vi "Lifting Position Calculations.vi"(0 "Limit switch 4":bool, 1 "position":enum16{"0", "1", "2", "3", "4"}(ring), 5 "Limit switch 3":bool, 7 "Limit switch 2":bool, 9 "Limit switch 1":bool, 11 "Bottom Limit switch":bool) -> (6 "Direction":enum16{"stop", "up", "down"}(ring), 10 "current position":dbl)   [LabVIEW 2014]
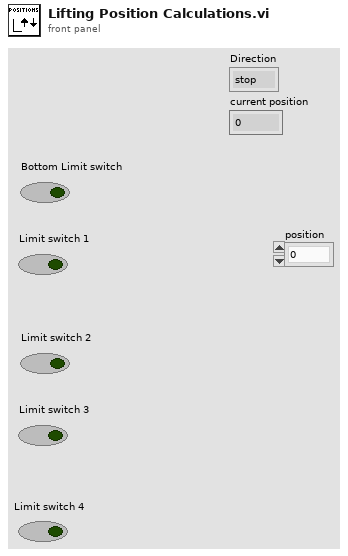
[diagram p1: front panel]
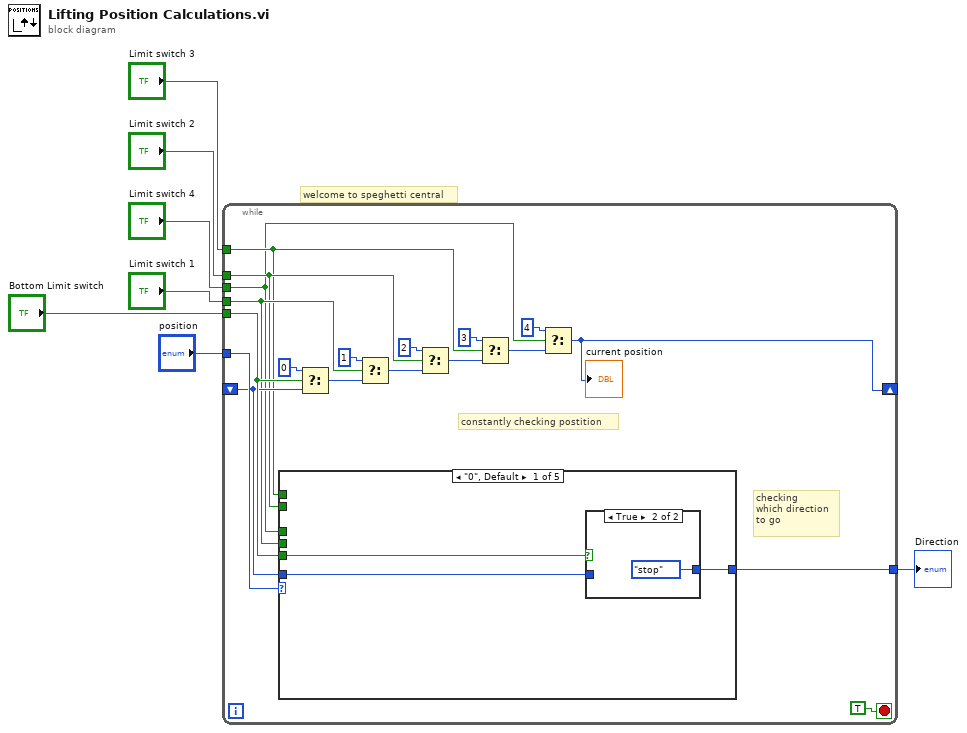
[diagram p0: block diagram]
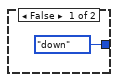
[diagram p2: hidden frame]
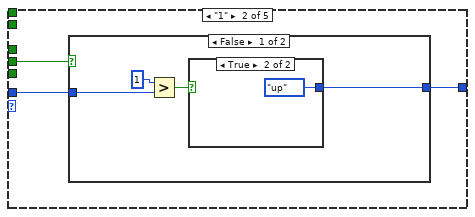
[diagram p3: hidden frame]
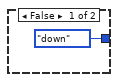
[diagram p4: hidden frame]
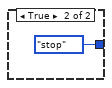
[diagram p5: hidden frame]
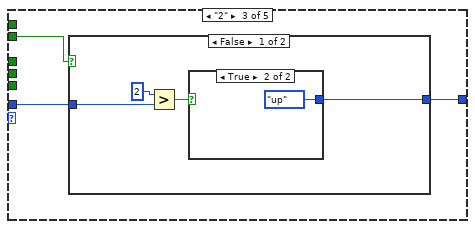
[diagram p6: hidden frame]
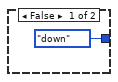
[diagram p7: hidden frame]
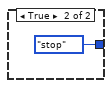
[diagram p8: hidden frame]
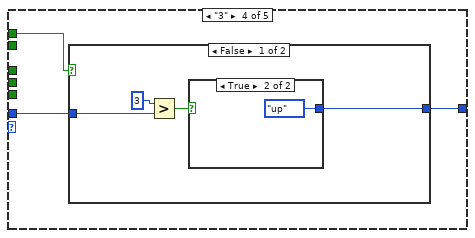
[diagram p9: hidden frame]
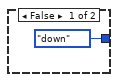
[diagram p10: hidden frame]
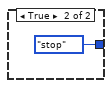
[diagram p11: hidden frame]
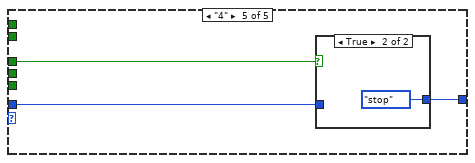
[diagram p12: hidden frame]
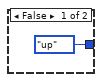
[diagram p13: hidden frame]
diagram:
  # "welcome to speghetti central"
  n1 = while {
    tunnel: "position" -> [w26]
    tunnel: [w25] -> w6
    tunnel: "Bottom Limit switch" -> [w13]
    tunnel: "Limit switch 1" -> [w11]
    tunnel: "Limit switch 2" -> [w10]
    tunnel: "Limit switch 3" -> [w9]
    tunnel: "Limit switch 4" -> [w8]
    shift-right: [w14] -> _
    shift-left: _ -> [w12]
    stop <- TRUE stop-if-true
    # "checking\nwhich direction\nto go"
    # "constantly checking postition"
    n2 = case shown="\"0\", Default" w26 {
      tunnel: [w29 w34 w44 w54 w64] -> w25
      tunnel: w13 -> [w28 _ _ _ _]
      tunnel: w11 -> [_ w33 _ _ _]
      tunnel: w10 -> [_ _ w43 _ _]
      tunnel: w9 -> [_ _ _ w53 _]
      tunnel: w8 -> [_ _ _ _ w63]
      tunnel: w12 -> [w27 w32 w42 w52 w62]
      frame "0", Default {
        n3 = case shown="True" w28 {
          tunnel: [enum16{"stop", "up", "down"}."down" ("Direction") enum16{"stop", "up", "down"}."stop" ("Direction")] -> w29
          tunnel: w27 -> [_ _]
          frame False {
          }
          frame True {
          }
        }
      }
      frame "1" {
        n4 = case shown="False" w33 {
          tunnel: [w38 enum16{"stop", "up", "down"}."stop" ("Direction")] -> w34
          tunnel: w32 -> [w35 _]
          frame False {
            n5 = Greater?(x=1, y=w35) -> (0:w36:bool)
            n6 = case shown="True" w36 {
              tunnel: [enum16{"stop", "up", "down"}."down" ("Direction") enum16{"stop", "up", "down"}."up" ("Direction")] -> w38
              frame False {
              }
              frame True {
              }
            }
          }
          frame True {
          }
        }
      }
      frame "2" {
        n7 = case shown="False" w43 {
          tunnel: [w48 enum16{"stop", "up", "down"}."stop" ("Direction")] -> w44
          tunnel: w42 -> [w45 _]
          frame False {
            n8 = Greater?(x=2, y=w45) -> (0:w47:bool)
            n9 = case shown="True" w47 {
              tunnel: [enum16{"stop", "up", "down"}."down" ("Direction") enum16{"stop", "up", "down"}."up" ("Direction")] -> w48
              frame False {
              }
              frame True {
              }
            }
          }
          frame True {
          }
        }
      }
      frame "3" {
        n10 = case shown="False" w53 {
          tunnel: [w58 enum16{"stop", "up", "down"}."stop" ("Direction")] -> w54
          tunnel: w52 -> [w55 _]
          frame False {
            n11 = Greater?(x=3, y=w55) -> (0:w57:bool)
            n12 = case shown="True" w57 {
              tunnel: [enum16{"stop", "up", "down"}."down" ("Direction") enum16{"stop", "up", "down"}."up" ("Direction")] -> w58
              frame False {
              }
              frame True {
              }
            }
          }
          frame True {
          }
        }
      }
      frame "4" {
        n13 = case shown="True" w63 {
          tunnel: [enum16{"stop", "up", "down"}."up" ("Direction") enum16{"stop", "up", "down"}."stop" ("Direction")] -> w64
          tunnel: w62 -> [_ _]
          frame False {
          }
          frame True {
          }
        }
      }
    }
    n14 = Select(t=0, s=w13, f=w12) -> (s? t:f=w18:i32)
    n15 = Select(t=1, s=w11, f=w18) -> (s? t:f=w17:i32)
    n16 = Select(t=2, s=w10, f=w17) -> (s? t:f=w16:i32)
    n17 = Select(t=3, s=w9, f=w16) -> (s? t:f=w15:i32)
    n18 = Select(t=4, s=w8, f=w15) -> (s? t:f=w14:i32)
    "current position" <- w14
  }
  "Direction" <- w6
